vi "mainActivity_应用程序.vi"() -> (0 "应用":T1(array[cluster]))   [LabVIEW 2014]
uses:
  R/manifest.vi
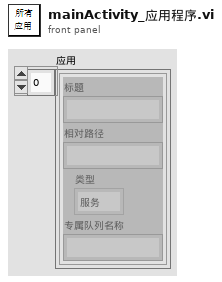
[diagram p1: front panel]
types:
  T1 = cluster{"标题":string, "相对路径":string, "类型":enum16{"服务", "活动"}, "专属队列名称":string}[]
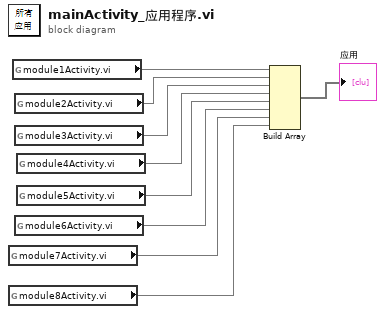
[diagram p0: block diagram]
diagram:
  n1 = global read "manifest.vi" "module7Activity.vi"() -> (w3)
  n2 = global read "manifest.vi" "module8Activity.vi"() -> (w2)
  n3 = global read "manifest.vi" "module1Activity.vi"() -> (w9)
  n4 = global read "manifest.vi" "module2Activity.vi"() -> (w8)
  n5 = global read "manifest.vi" "module3Activity.vi"() -> (w7)
  n6 = global read "manifest.vi" "module6Activity.vi"() -> (w4)
  n7 = global read "manifest.vi" "module4Activity.vi"() -> (w6)
  n8 = global read "manifest.vi" "module5Activity.vi"() -> (w5)
  n9 = Build Array(w9, w8, w7, w6, w5, w4, w3, w2) -> (→"应用":void[])
